vi "RadWag Self Calibration.vi"() -> ()   [LabVIEW 2016]
doc: "This VI runs internal calibration of balance. User is notified by boolean indicator if calibration was successfull. If some errors ocured during calibration processing user is notified by dialog message."
uses:
  <instrlib>/RadWag balances and scales/RadWag balances and scales.lvlib
panel:
  out "Calibration Successful":bool
  in  "VISA resource name":refnum<visa-resource-name>
  # "(c) 2014 Przemysłowy Instytut Automatyki i Pomiarów PIAP.  ALL RIGHTS RESERVED."
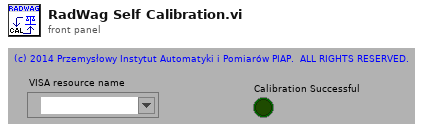
[diagram p1: front panel]
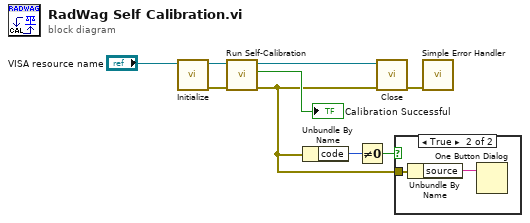
[diagram p0: block diagram]
diagram:
  n1 = call <instrlib>:"Initialize.vi"("VISA resource name"="VISA resource name") -> ("error out"=w8:errorcluster, "VISA resource name out"=w9:refnum<visa-resource-name>)  [unwired: 9 in]
  n2 = call <instrlib>:"Run Self-Calibration.vi"("error in (no error)"=w8, "VISA resource name"=w9) -> ("error out"=w1:errorcluster, "Calibration Successful"=→"Calibration Successful":bool, "VISA resource name out"=w6:refnum<visa-resource-name>)  [unwired: 7 in]
  n3 = Unbundle By Name(w1) -> ("code"=w3:i32)
  n4 = Not Equal To 0?(x=w3) -> (x != 0?=w2:bool)
  n5 = call <instrlib>:"Close.vi"("error in (no error)"=w1, "VISA resource name"=w6) -> ("error out"=w7:errorcluster)  [unwired: 9 in]
  n6 = case shown="True" w2 {
    tunnel: w1 -> [_ w11]
    frame False {
    }
    frame True {
      n7 = Unbundle By Name(w11) -> ("source"=w10:string)
      n8 = One Button Dialog(message=w10) -> ()  [unwired: 1 in, 1 out]
    }
  }
  n9 = call <vilib>:"Simple Error Handler.vi"("error in (no error)"=w7) -> ()  [unwired: 4 in, 5 out]
